vi "myRIO_BRig_RT_dataLC_Cue1_Probability_Switch_l2.vi"() -> (2 "output_Cue1_l2_First_Probability":i32)   [LabVIEW 2014]
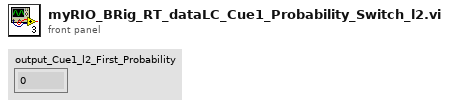
[diagram p1: front panel]
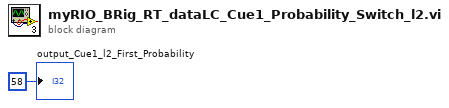
[diagram p0: block diagram]
diagram:
  "output_Cue1_l2_First_Probability" <- 58 ("output_iBlock")
